vi "Rectangle Sub-Parser.vi"(3 "error in (no error)":errorcluster, 5 "XML File Path In":path) -> (0 "error out":errorcluster, 1 "rects":T1[](array[typedef]), 2 "XML File Path Out":path)   [LabVIEW 2019]
uses:
  typedefs/Parsed Rect - Cluster.ctl
  <vilib>/Analysis/Matrix/Datatypes/RealMatrix.ctl
  <vilib>/Analysis/baseanly.llb/Real A x B.vi
  <vilib>/Analysis/NI_AALBase.lvlib
  <vilib>/Analysis/Matrix/NI_Matrix.lvlib
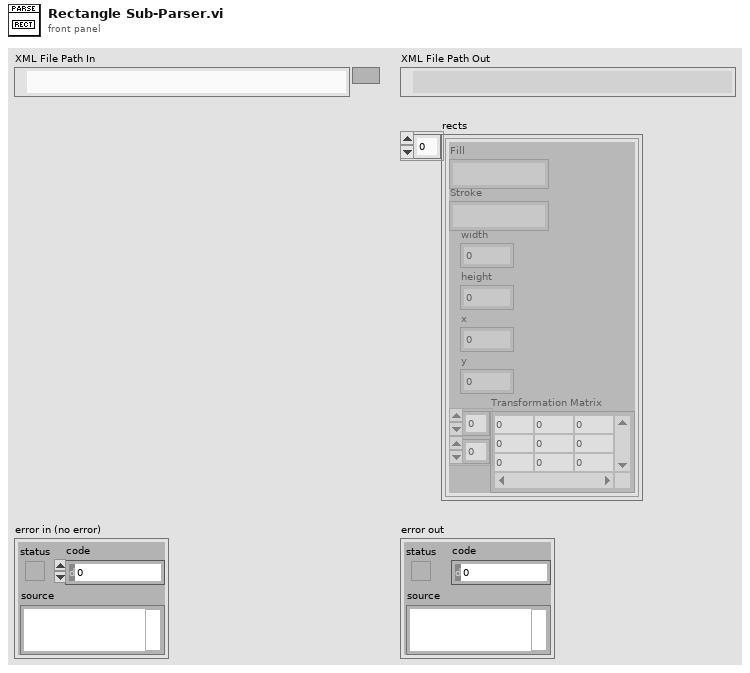
[diagram p1: front panel]
types:
  T1 = typedef "Parsed Rect - Cluster.ctl" = cluster{"Fill":string, "Stroke":string, "width":dbl, "height":dbl, "x":dbl, "y":dbl, "Transformation Matrix":T2}
  T2 = typedef "NI_Matrix.lvlib/RealMatrix.ctl" = dbl[][]
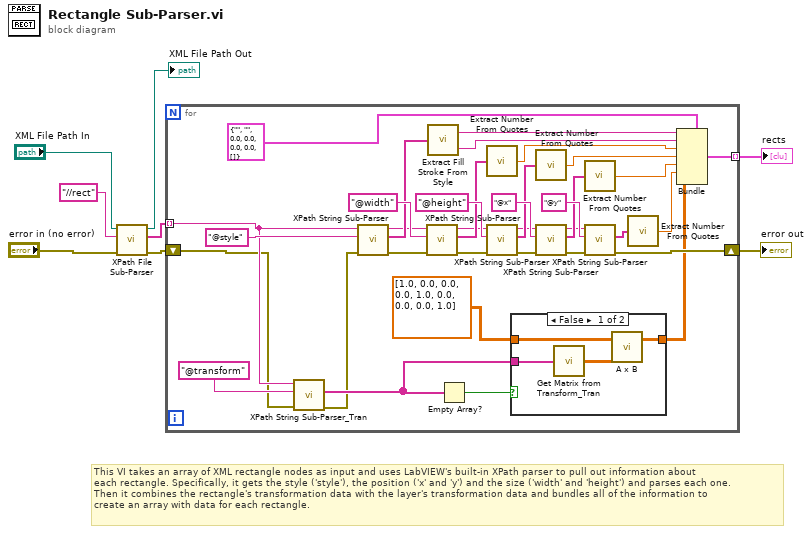
[diagram p0: block diagram]
diagram:
  # "This VI takes an array of XML rectangle nodes as input and uses LabVIEW's built-in XPath parser to pull out information about \neach rectangle. Specifically, it gets the style ('style'), the position ('x' and 'y') and the size ('width' and 'height') and parses each one.\nThen it combines the rectangle's transformation data with the layer's transformation data and bundles all of the information to\ncreate an array with data for each rectangle."
  n1 = call "XPath File Sub-Parser.vi"("error in (no error)"="error in (no error)", "XPath Expression"="//rect" ("XPath expression"), "XML File Path In"="XML File Path In") -> ("error out"=w3:errorcluster, "Array of Results"=w5:string[], "XML File Path Out"=→"XML File Path Out":path)  [unwired: 6 in]
  n2 = for {
    tunnel: w5 -> [w17] mode=indexing
    shift-right: [w34] -> w8
    shift-left: w3 -> [w10]
    tunnel: [w33] -> w1 mode=indexing
    n3 = call "XPath String Sub-Parser_Tran.vi"("error in (no error)"=w10, "XPath expression"="@transform", "XML String"=w17) -> ("error out"=w9:errorcluster, "Array of Results"=w14:string[])  [unwired: 6 in, 1 out]
    n4 = call "XPath String Sub-Parser.vi"("error in (no error)"=w9, "XPath expression"="@style", "XML String In"=w17) -> ("error out"=w41:errorcluster, "Array of Results"=w26:string[], "XML String Out"=w21:string)  [unwired: 6 in]
    n5 = call "XPath String Sub-Parser.vi"("error in (no error)"=w41, "XPath expression"="@width", "XML String In"=w21) -> ("error out"=w40:errorcluster, "Array of Results"=w25:string[], "XML String Out"=w20:string)  [unwired: 6 in]
    n6 = call "Extract Fill Stroke From Style.vi"("Array of Results"=w26) -> ("Fill"=w31:string, "Stroke"=w30:string)
    n7 = Empty Array?(array=w14) -> (empty?=w15:bool)
    n8 = call "Extract Number From Quotes.vi"("Array of Results"=w25) -> ("Numeric"=w27:dbl)
    n9 = call "XPath String Sub-Parser.vi"("error in (no error)"=w40, "XPath expression"="@height", "XML String In"=w20) -> ("error out"=w39:errorcluster, "Array of Results"=w24:string[], "XML String Out"=w19:string)  [unwired: 6 in]
    n10 = case shown="False" w15 {
      tunnel: [w47 w48] -> w12
      tunnel: w14 -> [w45 _]
      tunnel: T2 [[1.0, 0.0, 0.0], [0.0, 1.0, 0.0], [0.0, 0.0, 1.0]] ("Transformation Matrix") -> [w44 w48]
      frame False {
        n11 = call "Get Matrix from Transform_Tran.vi"("Transform Attributes"=w45) -> ("Matrix"=w46:T2)
        n12 = call-poly <vilib>:"A x B.vi"("B"=w46, "A"=w44) -> ("A x B"=w47:T2)  [unwired: 1 out]
      }
      frame True {
      }
    }
    n13 = call "Extract Number From Quotes.vi"("Array of Results"=w24) -> ("Numeric"=w32:dbl)
    n14 = call "XPath String Sub-Parser.vi"("error in (no error)"=w39, "XPath expression"="@x", "XML String In"=w19) -> ("error out"=w36:errorcluster, "Array of Results"=w23:string[], "XML String Out"=w18:string)  [unwired: 6 in]
    n15 = call "Extract Number From Quotes.vi"("Array of Results"=w23) -> ("Numeric"=w28:dbl)
    n16 = call "XPath String Sub-Parser.vi"("error in (no error)"=w36, "XPath expression"="@y", "XML String In"=w18) -> ("error out"=w34:errorcluster, "Array of Results"=w22:string[])  [unwired: 6 in, 1 out]
    n17 = call "Extract Number From Quotes.vi"("Array of Results"=w22) -> ("Numeric"=w29:dbl)
    n18 = Bundle(cluster=T1 {"Fill"="", "Stroke"="", "width"=0.0, "height"=0.0, "x"=0.0, "y"=0.0, "Transformation Matrix"=[]}, "Fill"=w31, "Stroke"=w30, "width"=w27, "height"=w32, "x"=w28, "y"=w29, "Transformation Matrix"=w12) -> (w33:T1)
  }
  "error out" <- w8
  "rects" <- w1
